vi "FdxCmdTMSetOptionsCvi.vi"(8 "error in":errorcluster, 9 "TMSetOptions":T1, 10 "TMHandle":u32, 11 "InstrumentHandle":u32) -> (0 "error out":errorcluster, 2 "TMHandleOut":u32, 3 "InstrumentHandle Out":u32)   [LabVIEW 2020, in "AIM664LV.lvlib"]
doc: "This function is used to configure the Time Manager options. It can be called while the Time Manager is running."
uses:
  AIM664LV.lvlib
  AFDX_LibraryAdmin/FdxGlobalDllPath.vi
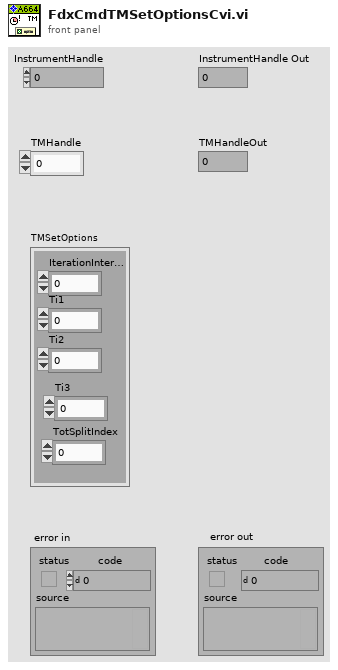
[diagram p1: front panel]
types:
  T1 = cluster{"IterationInterval":u32, "Ti1":u32, "Ti2":u32, "Ti3":u32, "TotSplitIndex":u8}
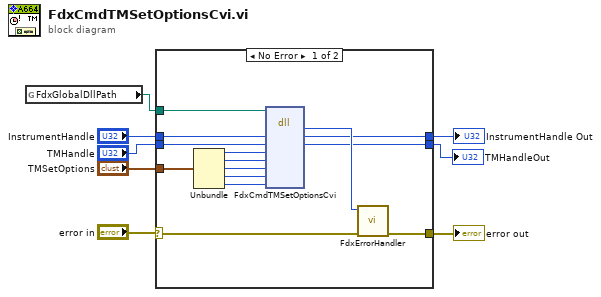
[diagram p0: block diagram]
diagram:
  n1 = global read "FdxGlobalDllPath.vi" "FdxGlobalDllPath"() -> (w6:path)
  n2 = case shown="No Error" "error in" {
    selector: "error in" -> [w21 w25]
    tunnel: [w22 w25] -> w8
    tunnel: w6 -> [w14 _]
    tunnel: [w13 w24] -> w5
    tunnel: "InstrumentHandle" -> [w12 w24]
    tunnel: "TMHandle" -> [w11 w23]
    tunnel: "TMSetOptions" -> [w10 _]
    tunnel: [w9 w23] -> w1
    frame No Error {
      n3 = Unbundle(w10) -> ("IterationInterval"=w19:u32, "Ti1"=w18:u32, "Ti2"=w17:u32, "Ti3"=w16:u32, "TotSplitIndex"=w15:u8)
      n4 = dll-call lib="aim_fdx.19.dll" fn="FdxCmdTMSetOptionsCvi"(path in=w14, "InstrumentHandle"=w12, "TMHandle"=w11, "IterationInterval"=w19, "Ti1"=w18, "Ti2"=w17, "Ti3"=w16, "TotSplitIndex"=w15) -> ("status"=w20:i32, "InstrumentHandle"=w13:u32, "TMHandle"=w9:u32)  [unwired: 7 in, 2 out]
      n5 = call "FdxErrorHandler.vi"("error in"=w21, "AIM Error"=w20) -> ("error out"=w22:errorcluster)  [unwired: 9 in]
    }
    frame Error {
    }
  }
  "error out" <- w8
  "InstrumentHandle Out" <- w5
  "TMHandleOut" <- w1
